vi "Emballage_BDD_indice_A_1.vi"(10 "NbrDeCar.":string="1", 11 "indiceLettre":string) -> (3 "indiceAttenduNum":string)   [LabVIEW 2020]
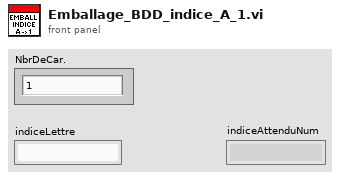
[diagram p1: front panel]
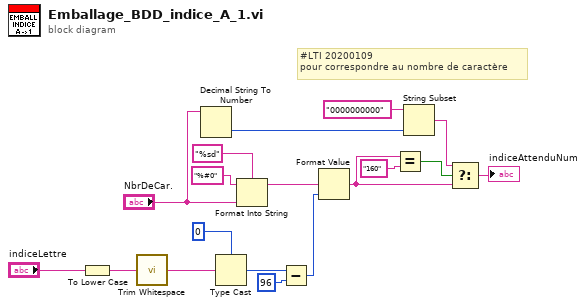
[diagram p0: block diagram]
diagram:
  # "#LTI 20200109\npour correspondre au nombre de caractère"
  n1 = To Lower Case(string="indiceLettre") -> (all lower case string=w8:string)
  n2 = call <vilib>:"Trim Whitespace.vi"("string"=w8) -> ("trimmed string"=w17:string)  [unwired: 1 in]
  n3 = Decimal String To Number(string="NbrDeCar.") -> (number=w1:i32)  [unwired: 2 in, 1 out]
  n4 = Type Cast(type=u8 0, x=w17) -> (*(type *) &x=w16:u8)
  n5 = Format Into String(format string="%sd" ("chaîne de format"), initial string="%#0" ("chaîne initiale"), "NbrDeCar.") -> (resulting string=w5:string)  [unwired: 1 in, 1 out]
  n6 = Subtract(x=w16, y=u8 96) -> (x-y=w14:u8)
  n7 = Format Value(format string=w5, value (0)=w14) -> (output string=w11:string)  [unwired: 1 in]
  n8 = Equal?(x=w11, y="160") -> (x = y?=w12:bool)
  n9 = String Subset(string="0000000000" ("chaîne"), length (rest)=w1) -> (substring=w3:string)  [unwired: 1 in]
  n10 = Select(t=w3, s=w12, f=w11) -> (s? t:f=→"indiceAttenduNum":string)
